vi "Get Unit Info.vi"(6 "路径":path, 8 "error in (no error)":errorcluster, 9 "Enable_User":bool, 10 "UserID":string, 11 "Serial Number":string="FZ01U1203247208660A000002C3") -> (0 "error out":errorcluster, 1 "Error Code":i64, 2 "strUnitInfo":string="<UnitInfo><UnitData><Name>SerialNumber</Name><Value>FZ01U1203247208660A000002C3</Value></UnitData><UnitData><Name>Check2Fail</Name><Value></Value></UnitData><UnitData><Name>MSUSN</Name><Value></Value></UnitData></UnitInfo>", 3 "Operation Success":bool, 4 "结果字符串":string, 5 "Station ID":string)   [LabVIEW 2017]
panel:
  in  "XML Prefix":string="<?xml version=\"1.0\" ?><GetUnitInfo xmlns=\"urn:GetUnitInfo-schema\" SerialNumber=\""
  in  "XML Suffix":string="\" />"
  in  "FFTester._Tester":refnum<k7>
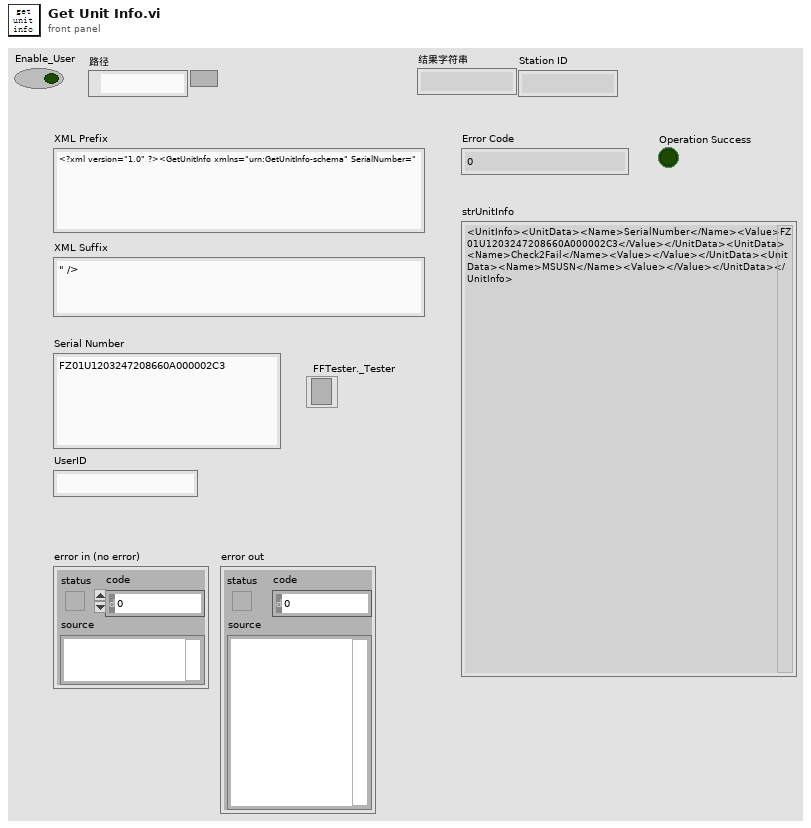
[diagram p1: front panel]
types:
  T1 = cluster{"strUnitInfo":string, "strStationName":string, "strUserID":string}
  T2 = enum16{"open", "replace", "create", "open or create", "replace or create", "replace or create with confirmation"}
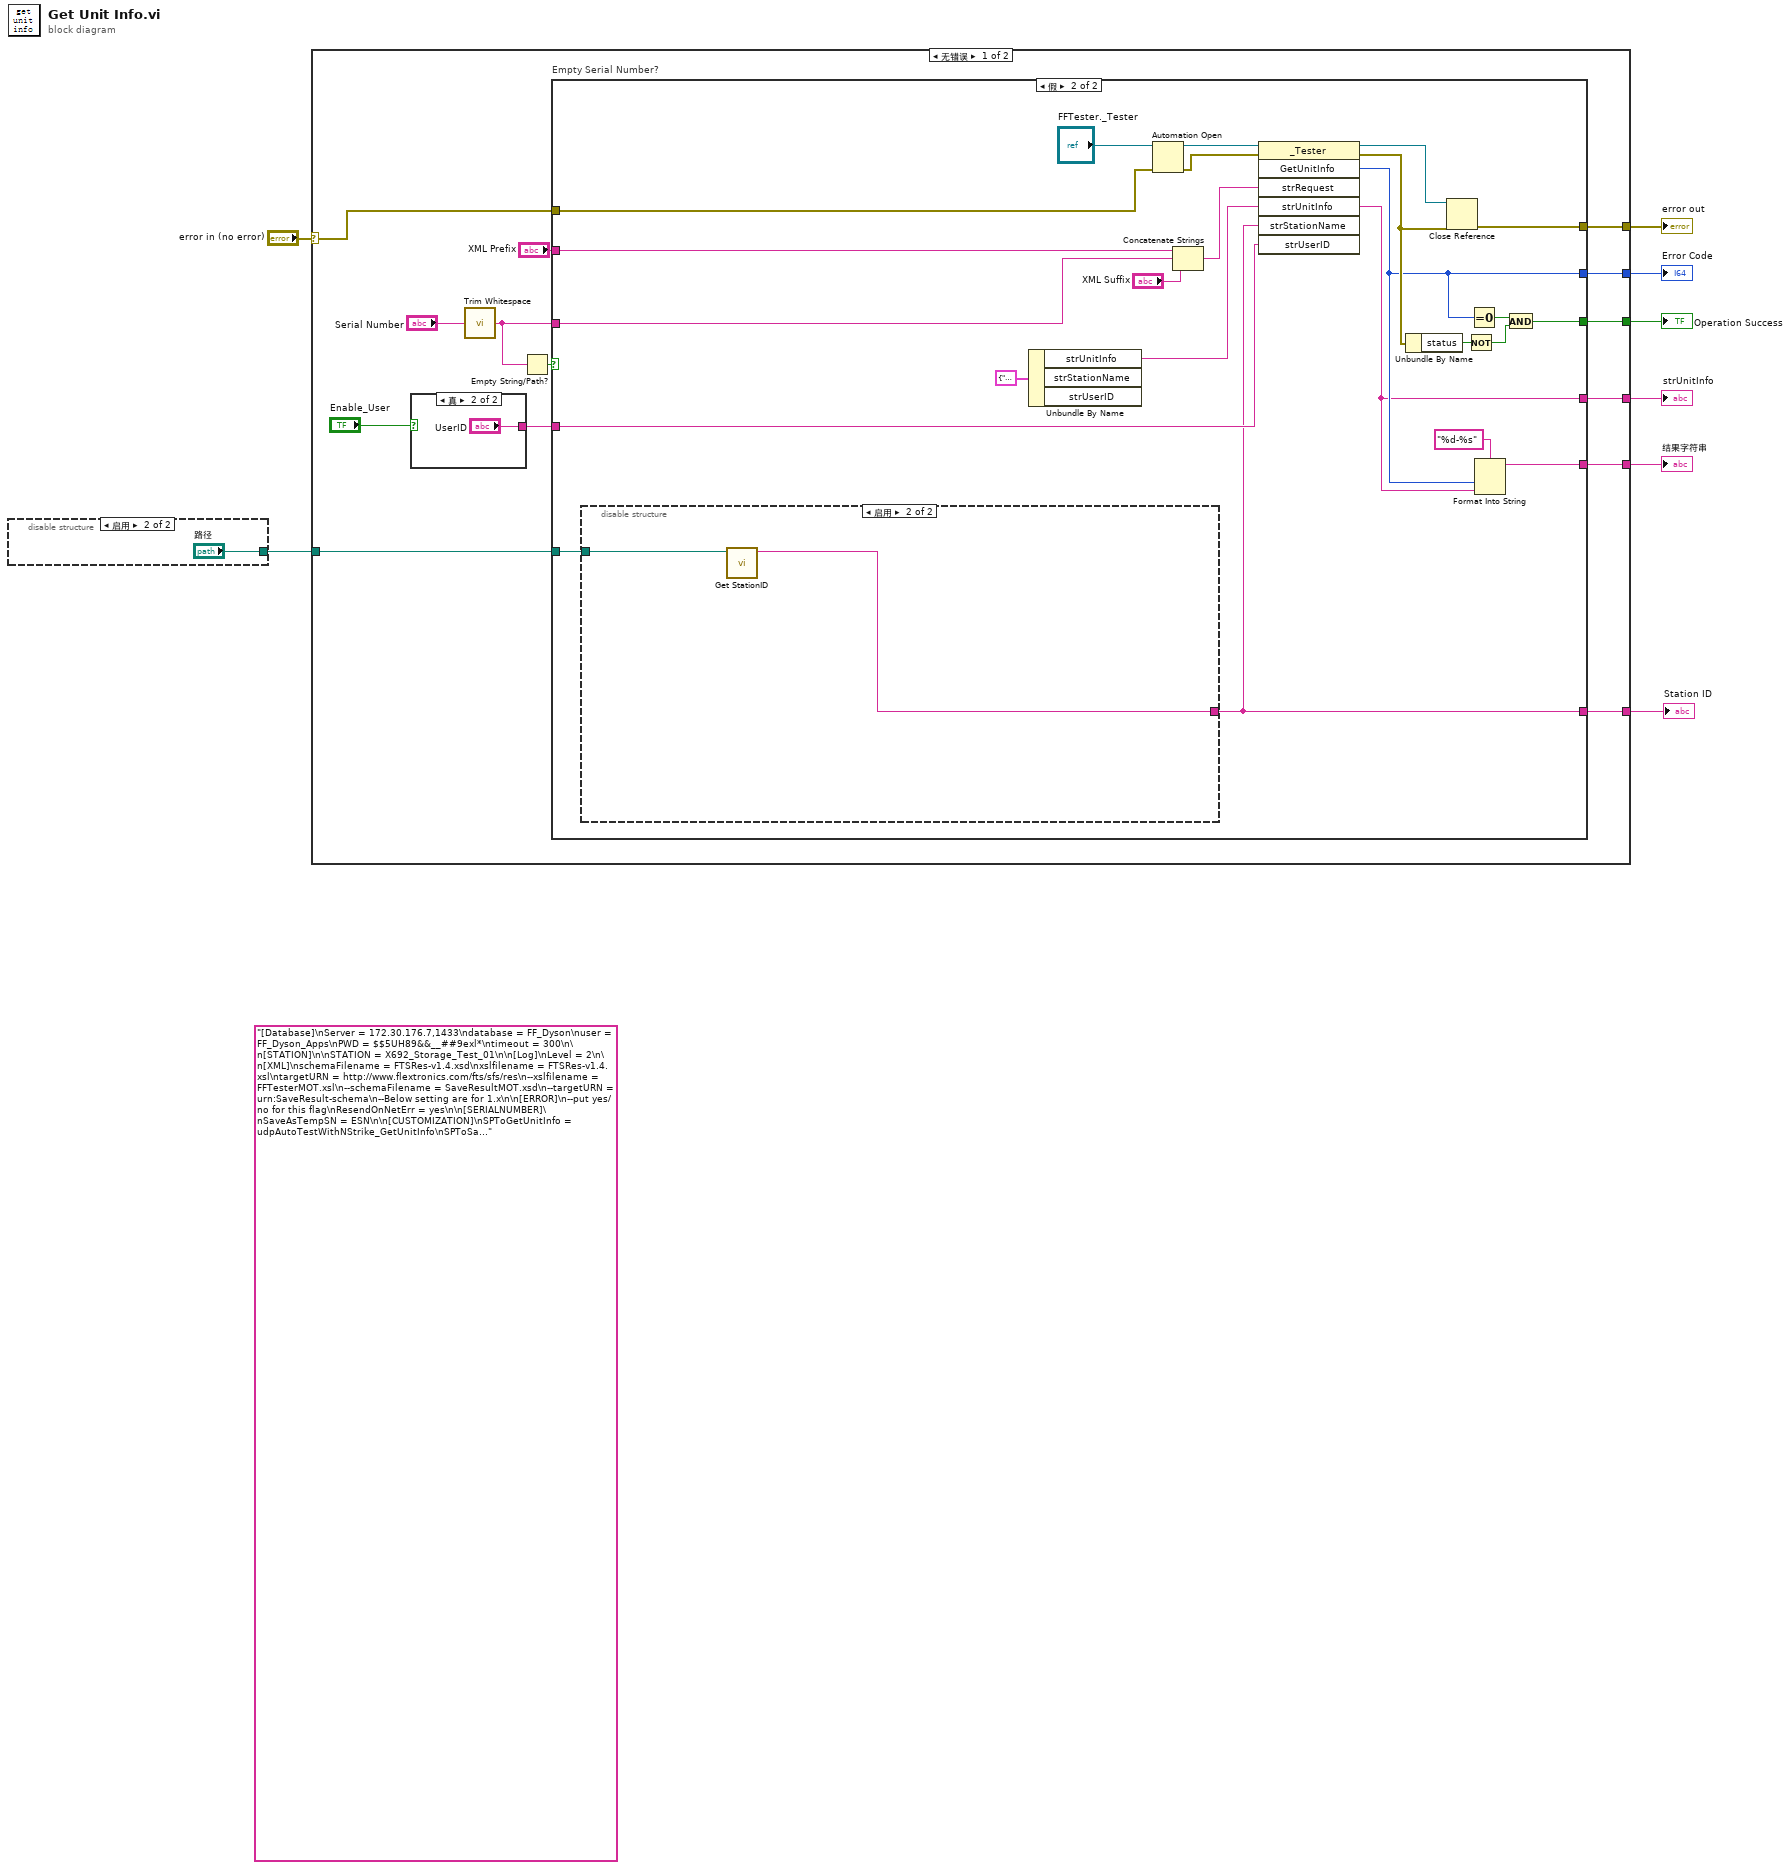
[diagram p0: block diagram]
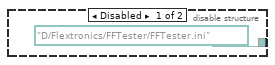
[diagram p2: hidden frame]
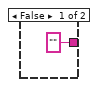
[diagram p3: hidden frame]
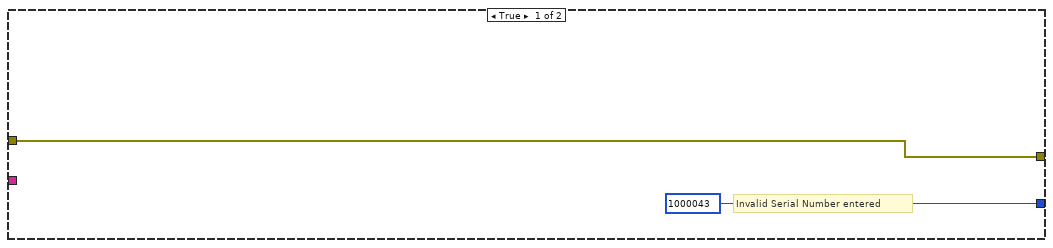
[diagram p4: hidden frame]
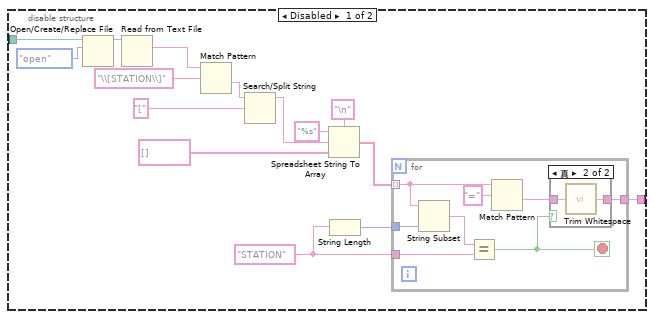
[diagram p5: hidden frame]
diagram:
  (unwired) "[Database]\nServer = 172.30.176.7,1433\ndatabase = FF_Dyson\nuser = FF_Dyson_Apps\nPWD = $$5UH89&&__##9exl*\ntimeout = 300\n\n[STATION]\n\nSTATION = X692_Storage_Test_01\n\n[Log]\nLevel = 2\n\n[XML]\nschemaFilename = FTSRes-v1.4.xsd\nxslfilename = FTSRes-v1.4.xsl\ntargetURN = http://www.flextronics.com/fts/sfs/res\n--xslfilename = FFTesterMOT.xsl\n--schemaFilename = SaveResultMOT.xsd\n--targetURN = urn:SaveResult-schema\n--Below setting are for 1.x\n\n[ERROR]\n--put yes/no for this flag\nResendOnNetErr = yes\n\n[SERIALNUMBER]\nSaveAsTempSN = ESN\n\n[CUSTOMIZATION]\nSPToGetUnitInfo = udpAutoTestWithNStrike_GetUnitInfo\nSPToSaveTestResult = udpDSN_SaveTestResult\n--SPToSaveTestResult = udpDSN_SaveTestResult_SkipFirstFail\nSPToGetProductStructure = \nSPToGenericFunction = \n\n[GENERICFUNCTIONSMAPPING]\n\n[SaveResultMethod]\nMethod = \n\n[Reporting-DB]\nServer = \ndatabase = \nuser = \nPWD = \n\n"
  n1 = disable-structure shown="启用" {
    disable-tunnel: [path "D:/Flextronics/FFTester/FFTester.ini" ("路径") "路径"] -> w2
    frame Disabled {
    }
    frame Enabled {
    }
  }
  n2 = case shown="无错误" "error in (no error)" {
    selector: "error in (no error)" -> [w18 w80]
    tunnel: [w23 _] -> w8
    tunnel: [w22 _] -> w5
    tunnel: [w21 w80] -> w7
    tunnel: [w16 _] -> w4
    tunnel: [w14 _] -> w3
    tunnel: w2 -> [w12 _]
    tunnel: [w11 _] -> w1
    frame No Error {
      n3 = case shown="真" "Enable_User" {
        tunnel: ["" ("UserID") "UserID"] -> w15
        frame False {
        }
        frame True {
        }
      }
      n4 = call <vilib>:"Trim Whitespace.vi"("string"="Serial Number") -> ("trimmed string"=w19:string)  [unwired: 1 in]
      n5 = Empty String/Path?(string/path=w19) -> (empty?=w17:bool)
      n6 = case "Empty Serial Number?" shown="假" w17 {
        tunnel: "XML Prefix" -> [_ w50]
        tunnel: [_ w32] -> w23
        tunnel: [i64 1000043 ("GetUnitInfo") w33] -> w22
        tunnel: [w28 w49] -> w21
        tunnel: w19 -> [_ w48]
        tunnel: w18 -> [w28 w38]
        tunnel: [_ w44] -> w16
        tunnel: w15 -> [_ w35]
        tunnel: [_ w31] -> w14
        tunnel: w12 -> [_ w30]
        tunnel: [_ w29] -> w11
        frame True {
          # "Invalid Serial Number entered"
        }
        frame False {
          n7 = disable-structure shown="启用" {
            disable-tunnel: w30 -> [w54 w79]
            disable-tunnel: [w53 w78] -> w29
            frame Disabled {
              w56 = "STATION"
              n8 = Open/Create/Replace File(file path (use dialog)=w54, operation (0:open)=T2."open" ("操作(0:open)")) -> (refnum out=w67:refnum<file>)  [unwired: 4 in, 2 out]
              n9 = Read from Text File(file (use dialog)=w67) -> (text=w62:string)  [unwired: 3 in, 3 out]
              n10 = Match Pattern(string=w62, regular expression="\\[STATION\\]") -> (after substring=w63:string)  [unwired: 1 in, 3 out]
              n11 = Search/Split String(string=w63, search string/char (-)="[") -> (substring before match=w60:string)  [unwired: 1 in, 2 out]
              n12 = Spreadsheet String To Array(delimiter (Tab)="\n" ("分隔符(Tab)"), format string="%s" ("格式字符串"), spreadsheet string=w60, array type (2D Dbl)=string[] []) -> (array=w57:string[])
              n13 = String Length(string=w56) -> (length=w55:i32)
              n14 = for {
                tunnel: w57 -> [w72] mode=indexing
                tunnel: w56 -> [w73]
                tunnel: w55 -> [w75]
                tunnel: [w68] -> w53
                stop <- w69 stop-if-true
                n15 = String Subset(string=w72, length (rest)=w75) -> (substring=w74:string)  [unwired: 1 in]
                n16 = Equal?(x=w74, y=w73) -> (x = y?=w69:bool)
                n17 = Match Pattern(string=w72, regular expression="=" ("正则表达式")) -> (after substring=w70:string)  [unwired: 1 in, 3 out]
                n18 = case shown="真" w69 {
                  tunnel: w70 -> [_ w77]
                  tunnel: [_ w76] -> w68
                  frame False {
                  }
                  frame True {
                    n19 = call <vilib>:"Trim Whitespace.vi"("string"=w77) -> ("trimmed string"=w76:string)  [unwired: 1 in]
                  }
                }
              }
            }
            frame Enabled {
              n20 = call "Get StationID.vi"("路径"=w79) -> ("Station ID"=w78:string)  [unwired: 10 in]
            }
          }
          n21 = Unbundle By Name(T1 {"strUnitInfo"="", "strStationName"="", "strUserID"=""} ("Additional Info (Blank)")) -> ("strUnitInfo"=w40:string)  [unwired: 2 out]
          n22 = Automation Open(error in (no error)=w38, Automation Refnum="FFTester._Tester") -> (Automation Refnum=w43:refnum<k7>, error out=w37:errorcluster)  [unwired: 2 in]
          n23 = Concatenate Strings(w50, w48, "XML Suffix") -> (w41:string)
          n24 = invoke on="调用节点" class="_Tester" method="GetUnitInfo"(reference=w43, error in=w37, "strRequest"=w41, "strUnitInfo"=w40, "strStationName"=w29, "strUserID"=w35) -> (reference out=w39:refnum<k7>, error out=w36:errorcluster, "GetUnitInfo"=w33:i32, "strUnitInfo"=w32:string)  [unwired: 1 in, 3 out]
          n25 = Unbundle By Name(w36) -> ("status"=w47:bool)
          n26 = Close Reference(reference=w39, error in (no error)=w36) -> (error out=w49:errorcluster)
          n27 = Not(x=w47) -> (.not. x?=w45:bool)
          n28 = Equal To 0?(x=w33) -> (x = 0?=w46:bool)
          n29 = Format Into String(format string="%d-%s" ("格式字符串"), w33, w32) -> (resulting string=w31:string)  [unwired: 2 in, 1 out]
          n30 = And(x=w46, y=w45) -> (x .and. y?=w44:bool)
        }
      }
    }
    frame Error {
    }
  }
  "strUnitInfo" <- w8
  "Error Code" <- w5
  "error out" <- w7
  "Operation Success" <- w4
  "结果字符串" <- w3
  "Station ID" <- w1
